vi "onDeserializeParameters.vi"(8 "error in (no error)":errorcluster, 10 "Variant":variant, 11 "Project in":refnum<class "Project.lvclass">) -> (0 "error out":errorcluster, 3 "Project out":refnum<class "Project.lvclass">)   [LabVIEW 2021, in "Bananas.lvlib" / "Project.lvclass"]
uses:
  Project.lvclass
  Project.lvclass/Project.ctl
  BananaPeel/BananaPeel.lvclass
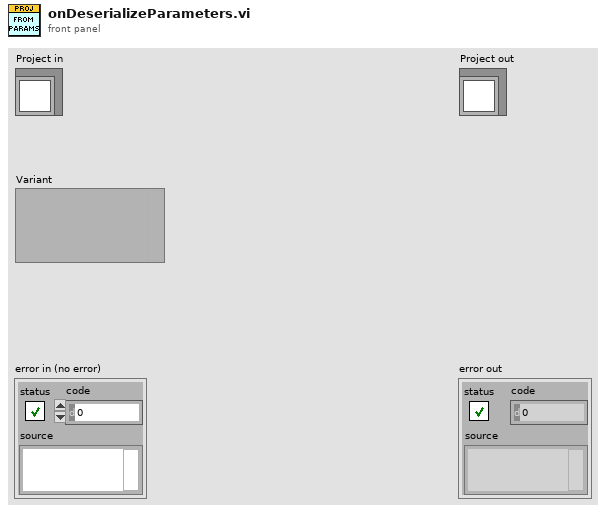
[diagram p1: front panel]
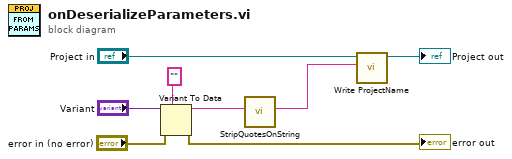
[diagram p0: block diagram]
diagram:
  n1 = Variant To Data(error in="error in (no error)", type="", Variant="Variant") -> (data=w3:string, error out=→"error out":errorcluster)
  n2 = call "StripQuotesOnString.vi"("String"=w3) -> ("Unquoted String"=w6:string)  [unwired: 10 in]
  n3 = call "Write ProjectName.vi"("ProjectName"=w6, "Project in"="Project in") -> ("Project out"=→"Project out":refnum<class "Project.lvclass">)  [unwired: 9 in]
